vi "Connect.vi"(8 "error in (no error)":errorcluster, 11 "N5745A in":refnum<class "5745A.lvclass">) -> (0 "error out":errorcluster, 3 "N5745A out":refnum<class "5745A.lvclass">)   [LabVIEW 2018, in "5745A.lvlib" / "5745A.lvclass"]
doc: "This Override method initializes communication with N5745A instrument."
uses:
  5745A.lvclass
  5745A.lvclass/5745A.ctl
  builds/Power_Supply.lvlibp/Power Supply.lvclass
  C:/Users/Ron.Dexter.LUMINARTECH/Desktop/builds/Power_Supply.lvlibp/Power Supply.lvclass
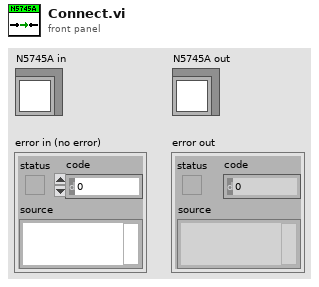
[diagram p1: front panel]
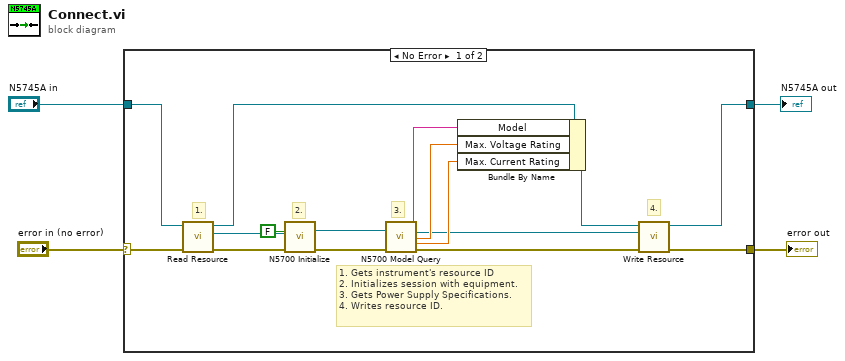
[diagram p0: block diagram]
diagram:
  n1 = case shown="No Error" "error in (no error)" {
    selector: "error in (no error)" -> [w16 w21]
    tunnel: "N5745A in" -> [w15 w22]
    tunnel: [w9 w22] -> w3
    tunnel: [w7 w21] -> w2
    frame No Error {
      # "1. Gets instrument's resource ID\n2. Initializes session with equipment.\n3. Gets Power Supply Specifications.\n4. Writes resource ID."
      # "4."
      # "3."
      # "2."
      # "1."
      n2 = call "Read Resource.vi"("error in"=w16, "Power Supply in"=w15) -> ("error out"=w19:errorcluster, "Resource"=w20:refnum<visa-resource-name>, "Power Supply out"=w14:refnum<class "5745A.lvclass">)  [unwired: 7 in]
      n3 = call <instrlib>:"N5700 Initialize.vi"("VISA name"=w20, "ID Query (T)"=FALSE, "error in (no error)"=w19) -> ("VISA out"=w18:refnum<visa-resource-name>, "error out"=w17:errorcluster)  [unwired: 11 in]
      n4 = call <instrlib>:"N5700 Model Query.vi"("error"=w17, "VISA"=w18) -> ("error out"=w8:errorcluster, "Current Rating"=w13:dbl, "Voltage Rating"=w12:dbl, "VISA out"=w6:refnum<visa-resource-name>, "Model"=w11:string)  [unwired: 2 in]
      n5 = Bundle By Name(cluster=w14, "Model"=w11, "Max. Voltage Rating"=w12, "Max. Current Rating"=w13) -> (w10:refnum<class "5745A.lvclass">)
      n6 = call "Write Resource.vi"("error in"=w8, "Resource"=w6, "Power Supply in"=w10) -> ("error out"=w7:errorcluster, "Power Supply out"=w9:refnum<class "5745A.lvclass">)  [unwired: 7 in]
    }
    frame Error {
    }
  }
  "error out" <- w2
  "N5745A out" <- w3
